vi "PHN.vi"(8 "error in":errorcluster, 10 "System Number":string, 11 "Arduino":refnum<visa-resource-name>) -> (0 "error out":errorcluster, 3 "Arduino out":refnum<visa-resource-name>)   [LabVIEW 2024]
panel:
  out "Responses":string
  out "Command Array":string[](array[string])
  out "StartTime":string
  out "Amplitudes":string[](array[string])
  out "Frequencies":string[](array[string])
  out "Temp Nom":string[](array[string])
  out "Nom":string[][](array[string])
  out "Nominal Frequency":string
  in  "DC_SN":string
  out "IsSine":bool=TRUE
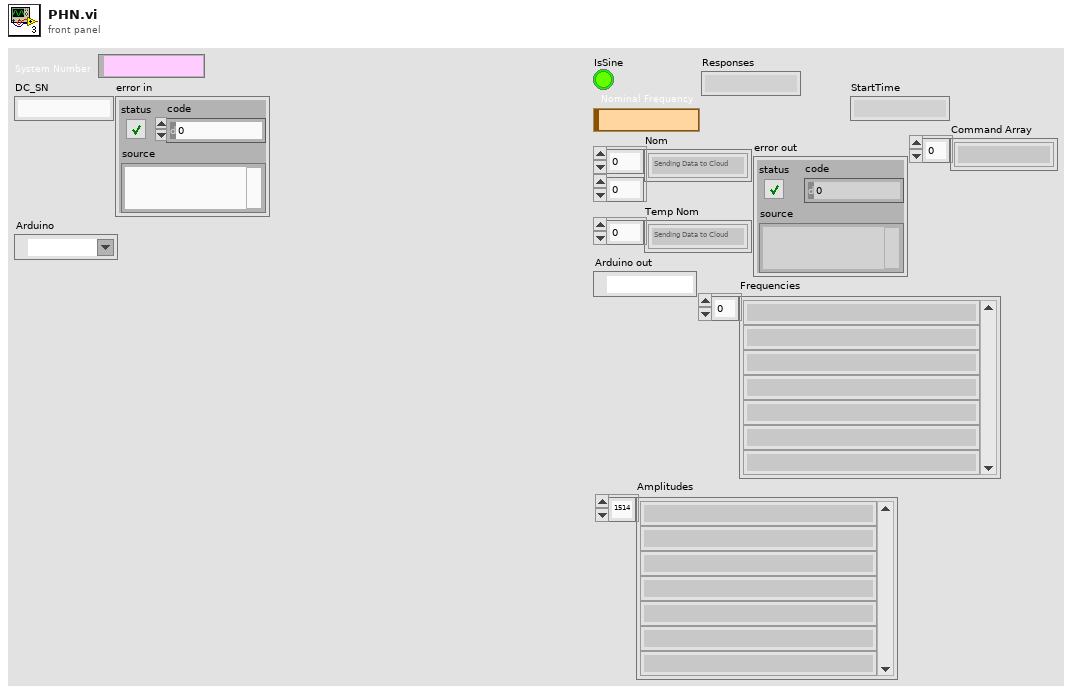
[diagram p1: front panel]
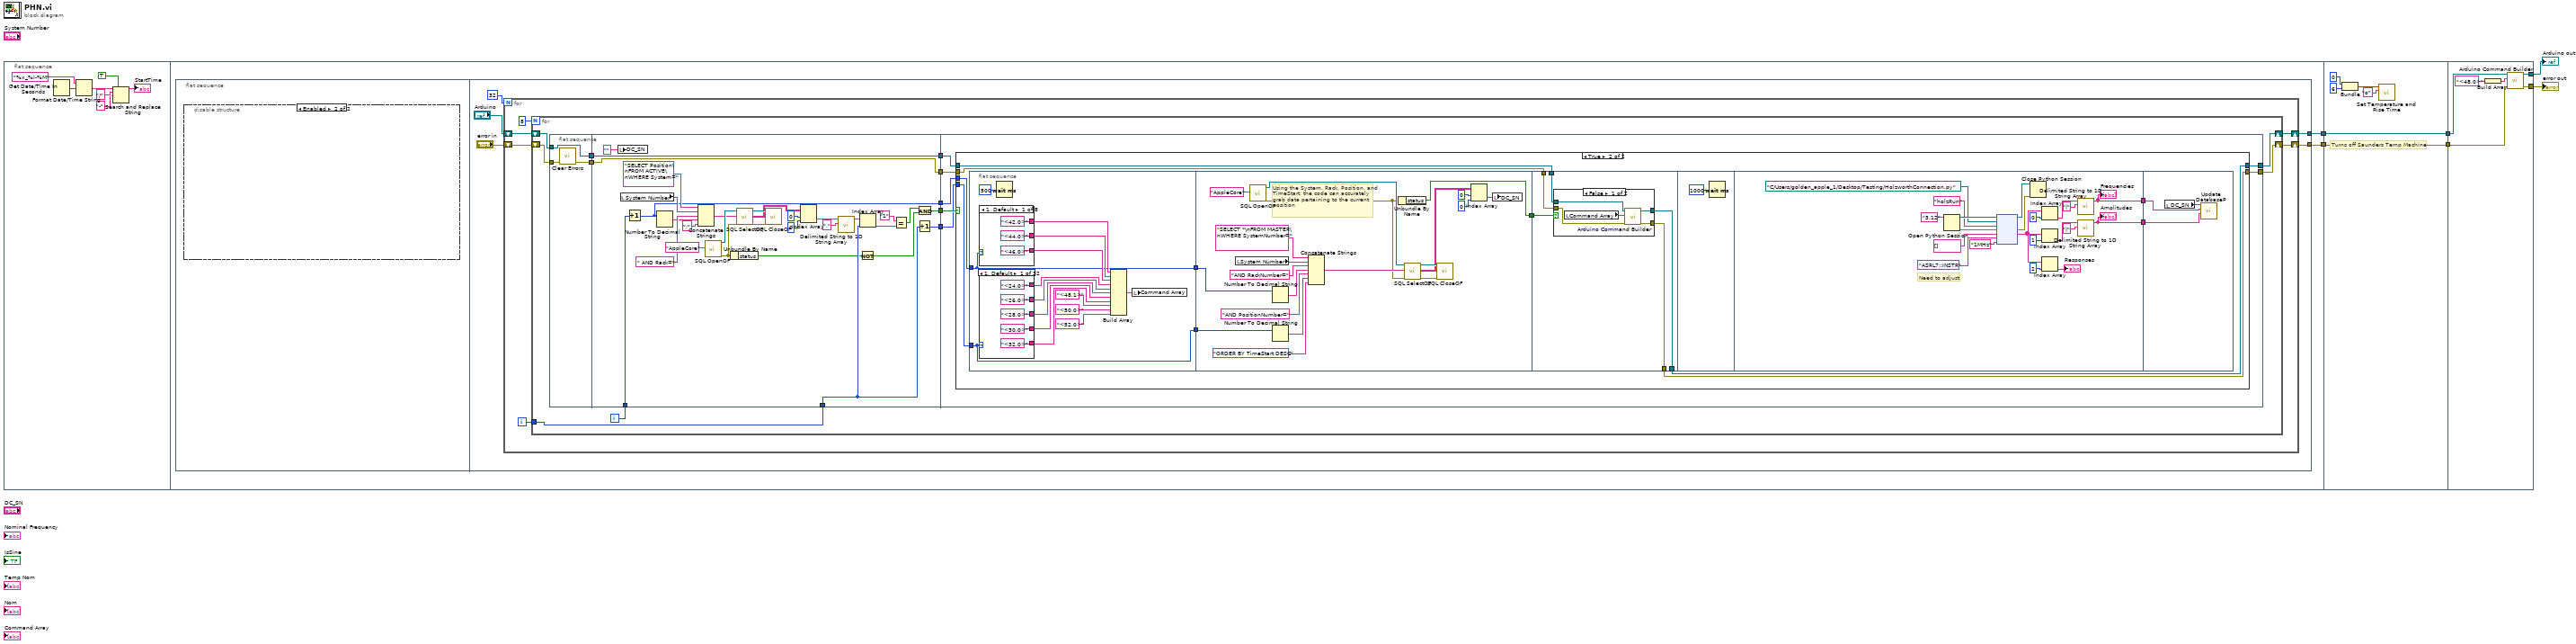
[diagram p0: block diagram]
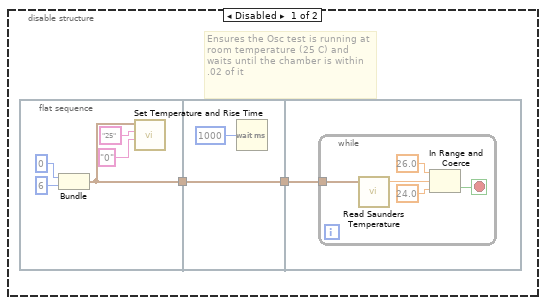
[diagram p2: hidden frame]
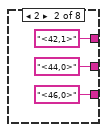
[diagram p4: hidden frame]
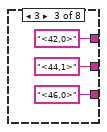
[diagram p5: hidden frame]
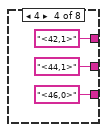
[diagram p6: hidden frame]
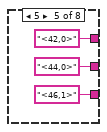
[diagram p7: hidden frame]
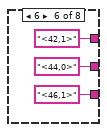
[diagram p8: hidden frame]
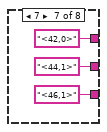
[diagram p9: hidden frame]
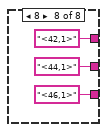
[diagram p10: hidden frame]
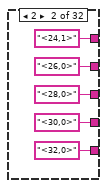
[diagram p11: hidden frame]
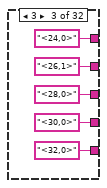
[diagram p12: hidden frame]
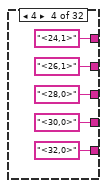
[diagram p13: hidden frame]
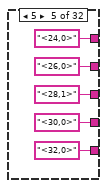
[diagram p14: hidden frame]
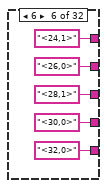
[diagram p15: hidden frame]
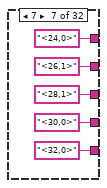
[diagram p16: hidden frame]
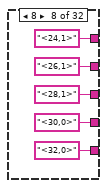
[diagram p17: hidden frame]
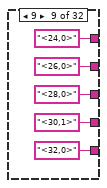
[diagram p18: hidden frame]
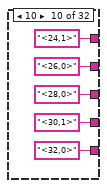
[diagram p19: hidden frame]
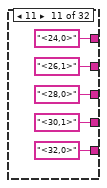
[diagram p20: hidden frame]
diagram:
  n1 = flat-sequence {
    tunnel: [w14] -> w6
    tunnel: [w15] -> w5
    tunnel: w5 -> [w364]
    tunnel: w6 -> [w365]
    tunnel: [w365] -> w3
    tunnel: [w364] -> w2
    tunnel: [w371] -> w4
    tunnel: w3 -> [w373]
    tunnel: w2 -> [w370]
    tunnel: [w372] -> w1
    frame #0 {
      n2 = Get Date/Time In Seconds() -> (seconds since 1Jan1904=w9:timestamp)
      n3 = Format Date/Time String(time format string (%c)="%x_%I-%M", seconds (now)=w9) -> (date/time string=w11:string)  [unwired: 1 in]
      n4 = Search and Replace String(replace all?=TRUE ("replace all? (F)"), input string=w11, search string="/", replace string="-" ("replace string (\"\")")) -> (result string=→"StartTime":string)  [unwired: 4 in, 3 out]
    }
    frame #1 {
      n5 = flat-sequence {
        tunnel: [w34] -> w14
        tunnel: [w33] -> w15
        frame #0 {
          n6 = disable-structure shown="Enabled" {
            frame Disabled {
              # "Ensures the Osc test is running at room temperature (25 C) and waits until the chamber is within .02 of it"
              n7 = flat-sequence {
                tunnel: [w19] -> w17
                tunnel: w17 -> [w24]
                tunnel: [w24] -> w16
                tunnel: w16 -> [w25]
                frame #0 {
                  n8 = Bundle(0, 6) -> (w19:cluster{i32, i32})  [unwired: 1 in]
                  n9 = call "Set Temperature and Rise Time.vi"("Slew Time String"="0", "Temperature String"="25", "Device"=w19) -> ()  [unwired: 3 in, 1 out]
                }
                frame #1 {
                  n10 = Wait (ms)(milliseconds to wait=u32 1000) -> ()  [unwired: 1 out]
                }
                frame #2 {
                  n11 = while {
                    tunnel: w25 -> [w30]
                    stop <- w26 stop-if-true
                    n12 = call "Read Saunders Temperature.vi"("Device"=w30) -> ("Temperature"=w29:dbl)  [unwired: 3 in, 1 out]
                    n13 = In Range and Coerce(upper limit=26.0, x=w29, lower limit=24.0) -> (In Range?=w26:bool)  [unwired: 1 out]
                  }
                }
              }
            }
            frame Enabled {
            }
          }
        }
        frame #1 {
          n14 = for {
            N: 32 -> [_]
            shift-right: [w37] -> w34
            shift-left: "error in" -> [w40]
            shift-right: [w36] -> w33
            shift-left: "Arduino" -> [w39]
            i -> [w38]
            n15 = for {
              N: 8 -> [_]
              shift-right: [w47] -> w37
              shift-left: w40 -> [w52]
              shift-right: [w42] -> w36
              shift-left: w39 -> [w51]
              tunnel: w38 -> [w50]
              i -> [w53]
              n16 = flat-sequence {
                tunnel: w52 -> [w57]
                tunnel: w51 -> [w56]
                tunnel: [w55] -> w46
                tunnel: [w56] -> w43
                tunnel: w53 -> [w68]
                tunnel: [w60] -> w54
                tunnel: w50 -> [w67]
                tunnel: [w66] -> w49
                tunnel: [w65] -> w48
                tunnel: w46 -> [w64]
                tunnel: [w64] -> w45
                tunnel: [w63] -> w44
                tunnel: w43 -> [w63]
                tunnel: w54 -> [w94]
                tunnel: w49 -> [w93]
                tunnel: w48 -> [w92]
                tunnel: [w88] -> w47
                tunnel: w45 -> [w91]
                tunnel: w44 -> [w90]
                tunnel: [w89] -> w42
                frame #0 {
                  n17 = call <vilib>:"Clear Errors.vi"("error in (no error)"=w57) -> ("error out"=w55:errorcluster)  [unwired: 5 in, 1 out]
                }
                frame #1 {
                  n18 = local write "DC_SN"("" ("DC.SN")) -> ()
                  n19 = local read "System Number"() -> (w73:string)
                  n20 = Increment(x=w68) -> (x+1=w66:i32)
                  n21 = Number To Decimal String(number=w66) -> (decimal integer string=w74:string)  [unwired: 1 in]
                  n22 = Concatenate Strings("SELECT Position\nFROM ACTIVE\nWHERE System=" ("SQL Query"), w73, " AND Rack=", w74, ";" ("string")) -> (w69:string)
                  n23 = call "SQL OpenOF.vi"("ConnectionString In"="AppleCore") -> ("Connection Out"=w80:refnum<k7>, "Error out"=w62:errorcluster)  [unwired: 17 in]
                  n24 = Unbundle By Name(w62) -> ("status"=w61:bool)
                  n25 = call "SQL SelectOF.vi"("Connection In"=w80, "SQL Query"=w69, "Error in (no error)"=w62) -> ("Connection Out"=w79:refnum<k7>, "Data"=w70:string[][], "Error out"=w78:errorcluster)  [unwired: 14 in]
                  n26 = call "SQL CloseOF.vi"("Connection In"=w79, "Error in (no error)"=w78) -> ()  [unwired: 17 in, 1 out]
                  n27 = Index Array(array=w70, index (row)=0 ("disabled index (row)"), index (col)=0 ("disabled index (col)")) -> (element=w87:string)
                  n28 = call <vilib>:"Delimited String to 1D String Array.vi"("delimiter"=",", "delimited string"=w87) -> ("string array"=w84:string[])  [unwired: 9 in]
                  n29 = Not(x=w61) -> (.not. x?=w58:bool)
                  n30 = Index Array(array=w84, index=w67) -> (element=w83:string)
                  n31 = Equal?(x="1", y=w83) -> (x = y?=w59:bool)
                  n32 = Increment(x=w67) -> (x+1=w65:i32)
                  n33 = And(x=w59, y=w58) -> (x .and. y?=w60:bool)
                }
                frame #2 {
                  n34 = case shown="True" w94 {
                    tunnel: w93 -> [_ w107]
                    tunnel: w92 -> [_ w106]
                    tunnel: w91 -> [w95 w103]
                    tunnel: w90 -> [w96 w102]
                    tunnel: [w96 w100] -> w89
                    tunnel: [w95 w99] -> w88
                    frame False {
                    }
                    frame True {
                      n35 = flat-sequence {
                        tunnel: w107 -> [w108]
                        tunnel: w106 -> [w109]
                        tunnel: [w109] -> w105
                        tunnel: [w108] -> w104
                        tunnel: w104 -> [w311]
                        tunnel: w105 -> [w326]
                        tunnel: [w309] -> w101
                        tunnel: w103 -> [w329]
                        tunnel: w102 -> [w330]
                        tunnel: w101 -> [w331]
                        tunnel: [w328] -> w100
                        tunnel: [w327] -> w99
                        tunnel: [w349] -> w98
                        tunnel: [w350] -> w97
                        tunnel: w98 -> [w363]
                        tunnel: w97 -> [w362]
                        frame #0 {
                          n36 = case shown="1, Default" w108 {
                            tunnel: ["<42,0>" ("string") "<42,1>" ("string") "<42,0>" ("string") "<42,1>" ("string") "<42,0>" ("string") "<42,1>" ("string") "<42,0>" ("string") "<42,1>" ("string")] -> w118
                            tunnel: ["<44,0>" ("string") "<44,0>" ("string") "<44,1>" ("string") "<44,1>" ("string") "<44,0>" ("string") "<44,0>" ("string") "<44,1>" ("string") "<44,1>" ("string")] -> w119
                            tunnel: ["<46,0>" ("string") "<46,0>" ("string") "<46,0>" ("string") "<46,0>" ("string") "<46,1>" ("string") "<46,1>" ("string") "<46,1>" ("string") "<46,1>" ("string")] -> w120
                            frame 1, Default {
                            }
                            frame 2 {
                            }
                            frame 3 {
                            }
                            frame 4 {
                            }
                            frame 5 {
                            }
                            frame 6 {
                            }
                            frame 7 {
                            }
                            frame 8 {
                            }
                          }
                          n37 = case shown="1, Default" w109 {
                            tunnel: ["<32,0>" ("string") "<32,0>" ("string") "<32,0>" ("string") "<32,0>" ("string") "<32,0>" ("string") "<32,0>" ("string") "<32,0>" ("string") "<32,0>" ("string") "<32,0>" ("string") "<32,0>" ("string") "<32,0>" ("string") "<32,0>" ("string") "<32,0>" ("string") "<32,0>" ("string") "<32,0>" ("string") "<32,0>" ("string") "<32,1>" ("string") "<32,1>" ("string") "<32,1>" ("string") "<32,1>" ("string") "<32,1>" ("string") "<32,1>" ("string") "<32,1>" ("string") "<32,1>" ("string") "<32,1>" ("string") "<32,1>" ("string") "<32,1>" ("string") "<32,1>" ("string") "<32,1>" ("string") "<32,1>" ("string") "<32,1>" ("string") "<32,1>" ("string")] -> w117
                            tunnel: ["<30,0>" ("string") "<30,0>" ("string") "<30,0>" ("string") "<30,0>" ("string") "<30,0>" ("string") "<30,0>" ("string") "<30,0>" ("string") "<30,0>" ("string") "<30,1>" ("string") "<30,1>" ("string") "<30,1>" ("string") "<30,1>" ("string") "<30,1>" ("string") "<30,1>" ("string") "<30,1>" ("string") "<30,1>" ("string") "<30,0>" ("string") "<30,0>" ("string") "<30,0>" ("string") "<30,0>" ("string") "<30,0>" ("string") "<30,0>" ("string") "<30,0>" ("string") "<30,0>" ("string") "<30,1>" ("string") "<30,1>" ("string") "<30,1>" ("string") "<30,1>" ("string") "<30,1>" ("string") "<30,1>" ("string") "<30,1>" ("string") "<30,1>" ("string")] -> w116
                            tunnel: ["<28,0>" ("string") "<28,0>" ("string") "<28,0>" ("string") "<28,0>" ("string") "<28,1>" ("string") "<28,1>" ("string") "<28,1>" ("string") "<28,1>" ("string") "<28,0>" ("string") "<28,0>" ("string") "<28,0>" ("string") "<28,0>" ("string") "<28,1>" ("string") "<28,1>" ("string") "<28,1>" ("string") "<28,1>" ("string") "<28,0>" ("string") "<28,0>" ("string") "<28,0>" ("string") "<28,0>" ("string") "<28,1>" ("string") "<28,1>" ("string") "<28,1>" ("string") "<28,1>" ("string") "<28,0>" ("string") "<28,0>" ("string") "<28,0>" ("string") "<28,0>" ("string") "<28,1>" ("string") "<28,1>" ("string") "<28,1>" ("string") "<28,1>" ("string")] -> w115
                            tunnel: ["<26,0>" ("string") "<26,0>" ("string") "<26,1>" ("string") "<26,1>" ("string") "<26,0>" ("string") "<26,0>" ("string") "<26,1>" ("string") "<26,1>" ("string") "<26,0>" ("string") "<26,0>" ("string") "<26,1>" ("string") "<26,1>" ("string") "<26,0>" ("string") "<26,0>" ("string") "<26,1>" ("string") "<26,1>" ("string") "<26,0>" ("string") "<26,0>" ("string") "<26,1>" ("string") "<26,1>" ("string") "<26,0>" ("string") "<26,0>" ("string") "<26,1>" ("string") "<26,1>" ("string") "<26,0>" ("string") "<26,0>" ("string") "<26,1>" ("string") "<26,1>" ("string") "<26,0>" ("string") "<26,0>" ("string") "<26,1>" ("string") "<26,1>" ("string")] -> w114
                            tunnel: ["<24,0>" ("string") "<24,1>" ("string") "<24,0>" ("string") "<24,1>" ("string") "<24,0>" ("string") "<24,1>" ("string") "<24,0>" ("string") "<24,1>" ("string") "<24,0>" ("string") "<24,1>" ("string") "<24,0>" ("string") "<24,1>" ("string") "<24,0>" ("string") "<24,1>" ("string") "<24,0>" ("string") "<24,1>" ("string") "<24,0>" ("string") "<24,1>" ("string") "<24,0>" ("string") "<24,1>" ("string") "<24,0>" ("string") "<24,1>" ("string") "<24,0>" ("string") "<24,1>" ("string") "<24,0>" ("string") "<24,1>" ("string") "<24,0>" ("string") "<24,1>" ("string") "<24,0>" ("string") "<24,1>" ("string") "<24,0>" ("string") "<24,1>" ("string")] -> w113
                            frame 1, Default {
                            }
                            frame 2 {
                            }
                            frame 3 {
                            }
                            frame 4 {
                            }
                            frame 5 {
                            }
                            frame 6 {
                            }
                            frame 7 {
                            }
                            frame 8 {
                            }
                            frame 9 {
                            }
                            frame 10 {
                            }
                            frame 11 {
                            }
                            frame 12 {
                            }
                            frame 13 {
                            }
                            frame 14 {
                            }
                            frame 15 {
                            }
                            frame 16 {
                            }
                            frame 17 {
                            }
                            frame 18 {
                            }
                            frame 19 {
                            }
                            frame 20 {
                            }
                            frame 21 {
                            }
                            frame 22 {
                            }
                            frame 23 {
                            }
                            frame 24 {
                            }
                            frame 25 {
                            }
                            frame 26 {
                            }
                            frame 27 {
                            }
                            frame 28 {
                            }
                            frame 29 {
                            }
                            frame 30 {
                            }
                            frame 31 {
                            }
                            frame 32 {
                            }
                          }
                          n38 = Wait (ms)(milliseconds to wait=u32 500 ("millisecond multiple")) -> ()  [unwired: 1 out]
                          n39 = Build Array(w118, w119, w120, w113, w114, w115, w116, w117, "<48,1>" ("string"), "<50,0>" ("string"), "<52,0>" ("string")) -> (w121:string[])
                          n40 = local write "Command Array"(w121) -> ()
                        }
                        frame #1 {
                          # "Using the System, Rack, Position, and TimeStart, the code can accurately grab data pertaining to the current position"
                          n41 = local read "System Number"() -> (w324:string)
                          n42 = call "SQL OpenOF.vi"("ConnectionString In"="AppleCore") -> ("Connection Out"=w314:refnum<k7>, "Error out"=w310:errorcluster)  [unwired: 17 in]
                          n43 = Number To Decimal String(number=w311) -> (decimal integer string=w322:string)  [unwired: 1 in]
                          n44 = Number To Decimal String(number=w326) -> (decimal integer string=w323:string)  [unwired: 1 in]
                          n45 = Concatenate Strings("SELECT *\nFROM MASTER\nWHERE SystemNumber=" ("SQL Query"), w324, "AND RackNumber=" ("string"), w322, "AND PositionNumber=" ("string"), w323, "ORDER BY TimeStart DESC" ("string")) -> (w325:string)
                          n46 = Unbundle By Name(w310) -> ("status"=w309:bool)
                          n47 = call "SQL SelectOF.vi"("Connection In"=w314, "SQL Query"=w325, "Error in (no error)"=w310) -> ("Connection Out"=w321:refnum<k7>, "Data"=w312:string[][], "Error out"=w320:errorcluster)  [unwired: 14 in]
                          n48 = call "SQL CloseOF.vi"("Connection In"=w321, "Error in (no error)"=w320) -> ()  [unwired: 17 in, 1 out]
                          n49 = Index Array(array=w312, index (row)=0, index (col)=0 ("disabled index (col)")) -> (element=w307:string)
                          n50 = local write "DC_SN"(w307) -> ()
                        }
                        frame #2 {
                          n51 = case shown="False" w331 {
                            tunnel: w330 -> [w336 w338]
                            tunnel: w329 -> [w335 w337]
                            tunnel: [w334 w338] -> w328
                            tunnel: [w333 w337] -> w327
                            frame False {
                              n52 = local read "Command Array"() -> (w332:string[])
                              n53 = call "Arduino Command Builder.vi"("error in"=w335, "Commands"=w332, "Arduino in"=w336) -> ("error out"=w333:errorcluster, "Arduino out"=w334:refnum<visa-resource-name>)  [unwired: 7 in]
                            }
                            frame True {
                            }
                          }
                        }
                        frame #3 {
                          n54 = Wait (ms)(milliseconds to wait=u32 1000 ("millisecond multiple")) -> ()  [unwired: 1 out]
                        }
                        frame #4 {
                          # "Need to adjust"
                          n55 = Open Python Session(python version="3.12" ("Python version")) -> (session out=w360:refnum<k35>, error out=w357:errorcluster)  [unwired: 2 in]
                          n56 = node ("Python Node")(w360, path "C:/Users/golden_apple_1/Desktop/Testing/HolzworthConnection.py" ("module path"), "holzRun" ("function name"), w357, string[] [] ("Python version"), "ASRL7::INSTR" ("Stop Point"), "1MHz" ("Stop Point")) -> (w359:refnum<k35>, w358:errorcluster, w346:string[])  [unwired: 2 in, 2 out]
                          n57 = Close Python Session(session in=w359, error in=w358) -> ()  [unwired: 1 out]
                          n58 = Index Array(array=w346, index=0) -> (element=w341:string)
                          n59 = Index Array(array=w346, index=1) -> (element=w340:string)
                          n60 = Index Array(array=w346, index=2) -> (element=→"Responses":string)
                          n61 = call <vilib>:"Delimited String to 1D String Array.vi"("delimiter"="|", "delimited string"=w341) -> ("string array"=w349:string[])  [unwired: 9 in]
                          "Frequencies" <- w349
                          n62 = call <vilib>:"Delimited String to 1D String Array.vi"("delimiter"="|", "delimited string"=w340) -> ("string array"=w350:string[])  [unwired: 9 in]
                          "Amplitudes" <- w350
                        }
                        frame #5 {
                          n63 = local read "DC_SN"() -> (w361:string)
                          n64 = call "Update DatabaseP.vi"("Amplitudes"=w362, "Frequencies"=w363, "DC_SN"=w361) -> ()  [unwired: 9 in]
                        }
                      }
                    }
                  }
                }
              }
            }
          }
        }
      }
    }
    frame #2 {
      # "Turns off Saunders Temp Machine"
      n65 = Bundle(0, 6) -> (w366:cluster{i32, i32})  [unwired: 1 in]
      n66 = call "Set Temperature and Rise Time.vi"("Temperature String"="o", "Device"=w366) -> ()  [unwired: 4 in, 1 out]
    }
    frame #3 {
      n67 = Build Array("<48,0>" ("string")) -> (w375:string[])
      n68 = call "Arduino Command Builder.vi"("error in"=w373, "Commands"=w375, "Arduino in"=w370) -> ("error out"=w372:errorcluster, "Arduino out"=w371:refnum<visa-resource-name>)  [unwired: 7 in]
    }
  }
  "error out" <- w1
  "Arduino out" <- w4
